vi "Scale Methane Flow.vi"(10 "Methane flow (cfm)":dbl) -> (1 "Methan Flow (cfm) out":dbl, 2 "Methane Voltage out":dbl)   [LabVIEW 2013]
doc: "This sub-VI scales desired methane flow in cubic-feet-per-minute to the appropriate voltage needed to\ncontrol the valves that control the methane flow."
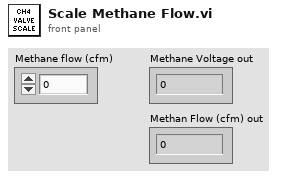
[diagram p1: front panel]
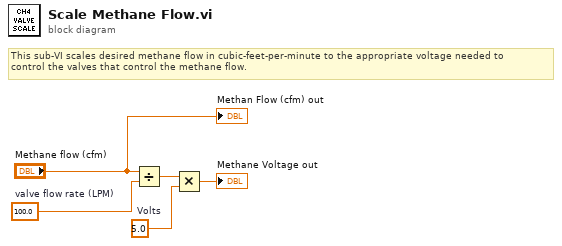
[diagram p0: block diagram]
diagram:
  w4 = 5.0  # Volts
  w2 = 100.0  # valve flow rate (LPM)
  # "This sub-VI scales desired methane flow in cubic-feet-per-minute to the appropriate voltage needed to\ncontrol the valves that control the methane flow."
  n1 = Divide(x="Methane flow (cfm)", y=w2) -> (x/y=w3:dbl)
  n2 = Multiply(x=w3, y=w4) -> (x*y=→"Methane Voltage out":dbl)
  "Methan Flow (cfm) out" <- "Methane flow (cfm)"
